vi "upload.file.vi"(8 "error in":errorcluster, 9 "timeout (ms)":i32=300000, 10 "File":path, 11 "Nominal Client in":refnum<class "Nominal Client.lvclass">) -> (0 "error out":errorcluster, 2 "Path to S3 File":string, 3 "Nominal Client out":refnum<class "Nominal Client.lvclass">)   [LabVIEW 2020, in "Nominal Client.lvclass"]
doc: "Uploads a file to S3. Intended for smaller files."
uses:
  Nominal Client.lvclass
  Nominal Client.lvclass/Nominal Client.ctl
  nominal types/workspace/workspace.lvclass/workspace.ctl
  <vilib>/JDP Science/JSONtext/LVClass Serializer/JSONtext LVClass Serializer.lvclass
  nominal types/workspace/workspace.lvclass
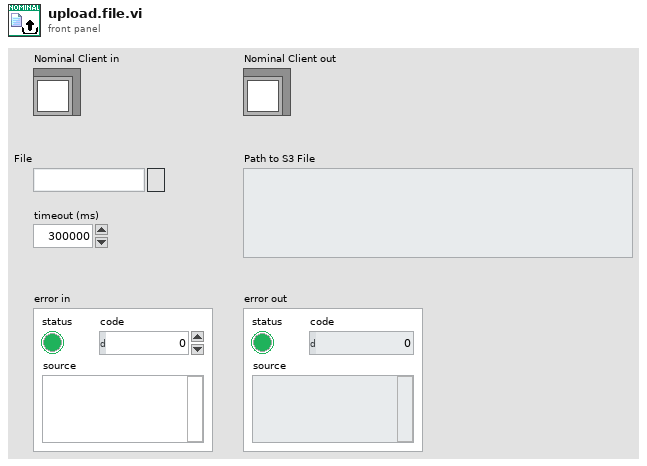
[diagram p1: front panel]
types:
  T1 = cluster{"override timeout":bool, "timeout override value (ms)":i32}
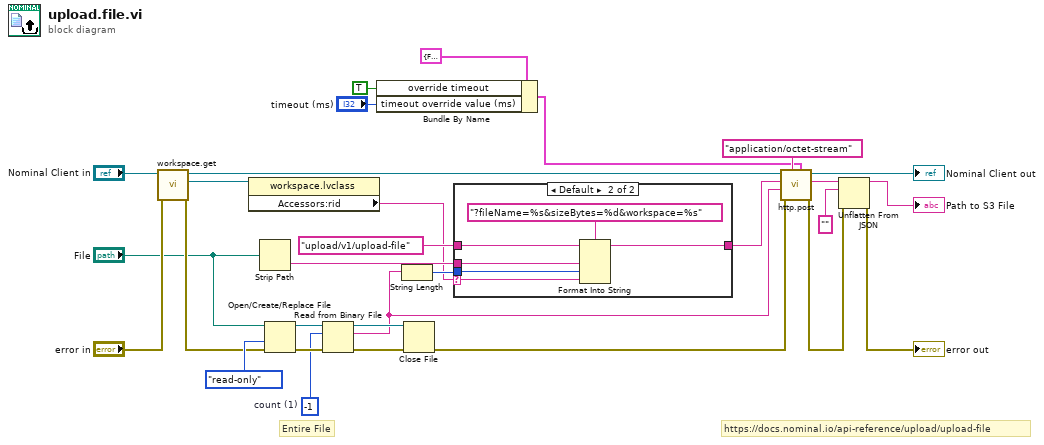
[diagram p0: block diagram]
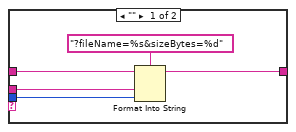
[diagram p2: hidden frame]
diagram:
  w24 = -1  # count (1)
  # "https://docs.nominal.io/api-reference/upload/upload-file"
  # "Entire File"
  n1 = call "workspace.get.vi"("error in"="error in", "Nominal Client in"="Nominal Client in") -> ("error out"=w8:errorcluster, "workspace"=w6:refnum<class "workspace.lvclass">, "Nominal Client out"=w11:refnum<class "Nominal Client.lvclass">)  [unwired: 7 in]
  n2 = property class="workspace.lvclass"(reference=w6) -> ("Accessors:rid"=w5:string)  [unwired: 1 in, 2 out]
  n3 = Strip Path(path="File") -> (name=w13:string)  [unwired: 1 out]
  n4 = Open/Create/Replace File(file path (use dialog)="File", error in=w8, access (0:read/write)=enum16{"read/write", "read-only", "write-only"}."read-only") -> (refnum out=w29:refnum<file>, error out=w28:errorcluster)  [unwired: 3 in, 1 out]
  n5 = Read from Binary File(8:w28, 10:w24, 11:w29) -> (0:w26:errorcluster, 2:w20:string, 3:w27:refnum<file>)  [unwired: 3 in, 1 out]
  n6 = Bundle By Name(cluster=T1 {"override timeout"=FALSE, "timeout override value (ms)"=300000} ("timeout override"), "override timeout"=TRUE, "timeout override value (ms)"="timeout (ms)") -> (w3:T1)
  n7 = String Length(string=w20) -> (length=w22:i32)
  n8 = Close File(refnum=w27, error in=w26) -> (error out=w23:errorcluster)  [unwired: 1 out]
  n9 = case shown="Default" w5 {
    selector: w5 -> [_ w36]
    tunnel: w22 -> [w34 w40]
    tunnel: "upload/v1/upload-file" ("Path") -> [w33 w39]
    tunnel: w13 -> [w32 w38]
    tunnel: [w31 w37] -> w10
    frame "" {
      n10 = Format Into String(format string="?fileName=%s&sizeBytes=%d" ("Path"), initial string=w33, w32, w34) -> (resulting string=w31:string)  [unwired: 1 in, 1 out]
    }
    frame Default {
      n11 = Format Into String(format string="?fileName=%s&sizeBytes=%d&workspace=%s" ("Path"), initial string=w39, w38, w40, w36) -> (resulting string=w37:string)  [unwired: 1 in, 1 out]
    }
  }
  n12 = call "http.post.vi"("timeout override"=w3, "Content Type"="application/octet-stream", "error in"=w23, "Request body"=w20, "Path"=w10, "Nominal Client in"=w11) -> ("error out"=w15:errorcluster, "Response"=w18:string, "Nominal Client out"=→"Nominal Client out":refnum<class "Nominal Client.lvclass">)  [unwired: 3 in]
  n13 = Unflatten From JSON(JSON string=w18, type and defaults="", error in (no error)=w15) -> (value=→"Path to S3 File":string, error out=→"error out":errorcluster)  [unwired: 4 in]
